vi "AutonomousGyro.vi"() -> (0 "Terminate":bool)   [LabVIEW 2015]
uses:
  <vilib>/Rock Robotics/WPI/DriverStation/WPI_DriverStationRobotMode2.ctl
  <vilib>/Rock Robotics/WPI/Solenoid/WPI_SolenoidValue.ctl
  Utilities/AutoVars.vi
  Utilities/MotorPositionGlobals.vi
  Utilities/ShiftGlobals.vi
  Utilities/VisionGlobals.vi
  Utilities/GlobalVisionVars.vi
  <vilib>/Rock Robotics/WPI/Solenoid/WPI_SolenoidSetEnum.vi
  navx-mxp/labview/navX Library v2/navX Library v2.lvlib
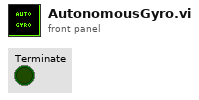
[diagram p1: front panel]
types:
  T1 = enum16{"WaitingForInput", "Driving", "TurnToTarget", "DriveMore", "Shoot", "End"}
  T2 = typedef "WPI_DriverStationRobotMode2.ctl" = enum16{"Autonomous Disabled", "Autonomous Enabled", "Teleop Disabled", "Teleop Enabled", "Disconnected", "Finish", "Test Disabled", "Test Enabled", "Emergency Stopped"}
  T3 = typedef "WPI_SolenoidValue.ctl" = enum16{"Off", "On", "Forward", "Reverse"}
  T4 = typedef "WPI_MotorControlDeviceRef.ctl" = cluster{"DeviceStatus":errorcluster, "Type":T5, "PWM":cluster{"PWM Channel":T6, "DeadBand":T7}, "CAN":cluster{"Device Number":u8, "Control Mode":T8, "Semaphore":T9, "Max Vout":dbl, "TalonSRX Control Mode":T10}, "Invert":bool}
  T5 = typedef "WPI_MotorControlType.ctl" = enum16{"PWM", "CAN", "CANTalonSRX"}
  T6 = typedef "FPGA_DIOPWMChannel.ctl" = enum8{"PWM 0", "PWM 1", "PWM 2", "PWM 3", "PWM 4", "PWM 5", "PWM 6", "PWM 7", "PWM 8", "PWM 9", "PWM MXP 0", "PWM MXP 1", "PWM MXP 2", "PWM MXP 3", "PWM MXP 4", "PWM MXP 5", "PWM MXP 6", "PWM MXP 7", "PWM MXP 8", "PWM MXP 9", "Invalid"}
  T7 = typedef "WPI_PWMDeadband.ctl" = cluster{"Name":string, "maxPositivePwm":i32, "minPositivePwm":i32, "centerPwm":i32, "maxNegativePwm":i32, "minNegativePwm":i32, "angularRange":u16}
  T8 = typedef "WPI_CANJaguar_ControlMode.ctl" = enum8{"Percent VBus", "Current", "Speed", "Position", "Voltage"}
  T9 = typedef "Semaphore RefNum" = refnum<k1>
  T10 = typedef "WPI_CANTalonSRX_APIControlMode.ctl" = enum8{"Percent VBus", "Speed", "Position", "Slave", "Unchanged / Invalid", "Voltage Compensation", "Current", "Motion Profile"}
  T11 = typedef "navX Library v2.lvlib/Z900_navX_DeviceTypeDef.ctl" = cluster{"Interface":cluster{"Protocol":T12, "Update Rate (4Hz-60Hz)":u8, "navX Open TypeDef":variant}, "Notify Packet":refnum<notifier>, "Loop VI Refnum":refnum<vi>, "Ready to Close Occurrence Refnum":refnum<k4>}
  T12 = typedef "navX Library v2.lvlib/Z900_navX_ProtocolTypeDef.ctl" = enum16{"SERIAL", "I2C", "SPI"}
  T13 = typedef "WPI_CANTalonSRX_GlobalStatus.ctl" = cluster{"Applied Throttle":dbl, "Module Enabled":bool, "CAN Error":errorcluster, "Closed Loop Error":dbl, "Forward Limit Switch Closed":bool, "Reverse Limit Switch Closed":bool, "Sensor Position":dbl, "Sensor Velocity":dbl, "Current":dbl, "Sticky Fault - Over Temp":bool, "Sticky Fault - Under Voltage":bool, "Sticky Fault - Forward Limit":bool, "Sticky Fault - Reverse Limit":bool, "Sticky Fault - Forward Soft Limit":bool, "Sticky Fault - Reverse Soft Limit":bool, "Brake is Enabled":bool, "Encoder Position":dbl, "Encoder Velocity":dbl, "Encoder Index Count":dbl, "Encoder A Pin State":bool, "Encoder B Pin State":bool, "Encoder Index Pin State":bool, "Analog In":dbl, "Analog In Velocity":dbl, "Temperature (C)":dbl, "Battery Voltage":dbl, "Control 5 Is Supported":bool, "Current Profile Slot Select":dbl, "Pos Div 8":bool, "Vel Div 4":bool, "Pulse Width Position":i32, "Pulse Width Velocity":i32, "Pulse Width Rise To Rise (us)":i32, "Pulse Width Rise To Fall (us)":i32, "Mot Prof Active Is Under Run":bool, "Mot Prof Active Has Under Run":bool, "Mot Prof Active Is Last":bool, "Mot Prof Active Velocity Only":bool, "Mot Prof Active Is Valid":bool, "Mot Prof Buffer Is Full":bool, "Mot Prof Active Profile Slot Select":i32, "Mot Prof NextID":i32, "Mot Prof Count":i32, "Mot Prof Active Velocity":dbl, "Mot Prof Active Position":dbl, "Mot Prof Output Enable":i32}
  T14 = typedef "WPI_DigitalOutputDevRef.ctl" = cluster{"DIO Channel":T15, "DevStatus":errorcluster}
  T15 = typedef "FPGA_DIOChannel.ctl" = enum8{"DIO 0", "DIO 1", "DIO 2", "DIO 3", "DIO 4", "DIO 5", "DIO 6", "DIO 7", "DIO 8", "DIO 9", "DIO MXP 0", "DIO MXP 1", "DIO MXP 2", "DIO MXP 3", "DIO MXP 4", "DIO MXP 5", "DIO MXP 6", "DIO MXP 7", "DIO MXP 8", "DIO MXP 9", "DIO MXP 10", "DIO MXP 11", "DIO MXP 12", "DIO MXP 13", "DIO MXP 14", "DIO MXP 15", "Invalid"}
  T16 = typedef "WPI_SolenoidDevRef.ctl" = cluster{"DevStatus":errorcluster, "Pneumatics Control Module":u8, "Forward Solenoid Channel":T17, "Reverse Solenoid Channel":T17}
  T17 = typedef "WPI_SolenoidChannel.ctl" = enum8{"Solenoid 0", "Solenoid 1", "Solenoid 2", "Solenoid 3", "Solenoid 4", "Solenoid 5", "Solenoid 6", "Solenoid 7", "Invalid"}
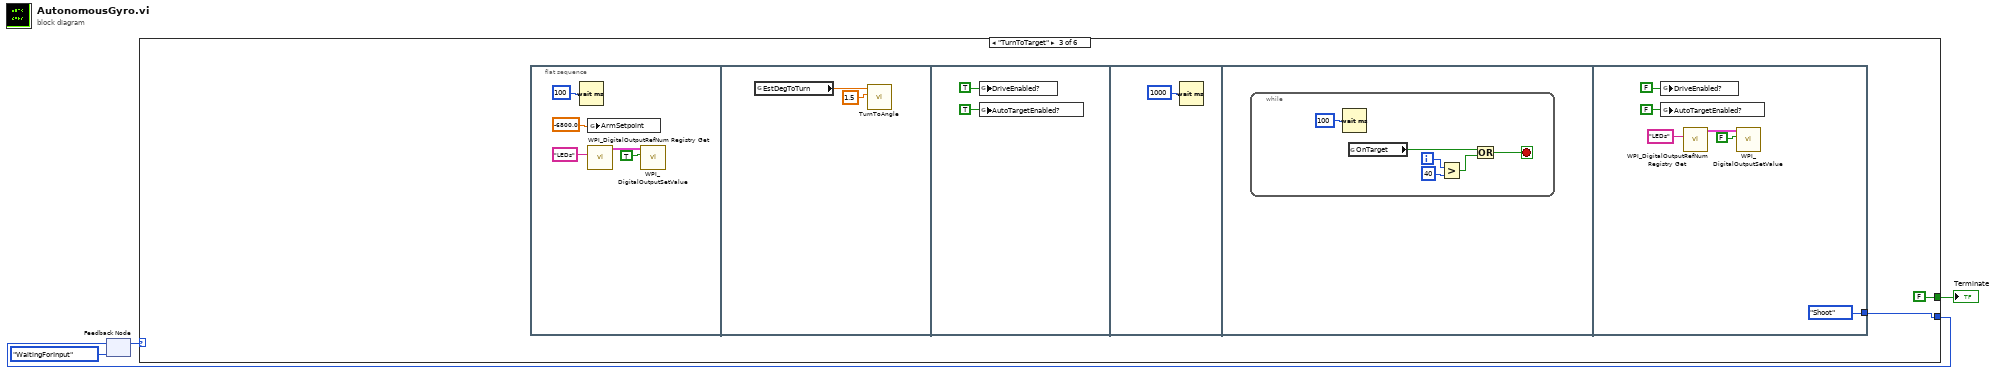
[diagram p0: block diagram]
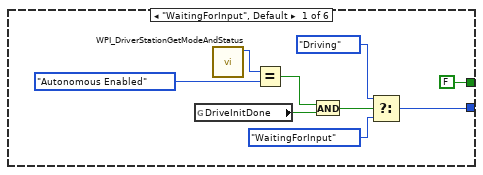
[diagram p2: hidden frame]
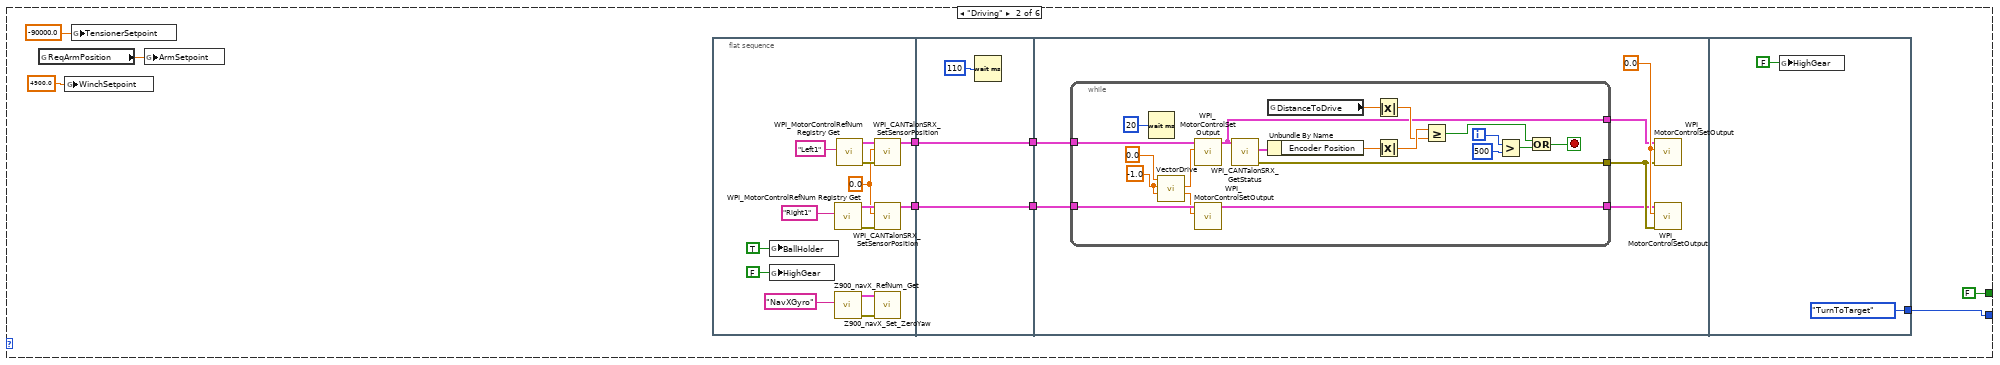
[diagram p3: hidden frame]
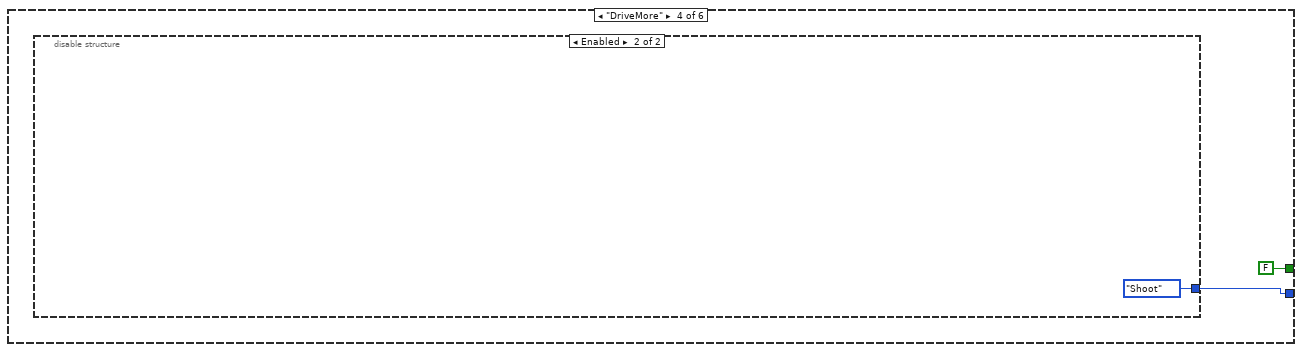
[diagram p4: hidden frame]
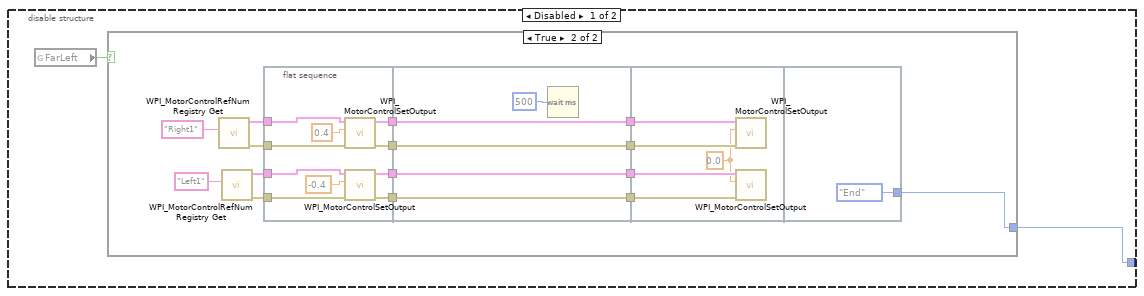
[diagram p5: hidden frame]
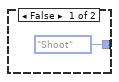
[diagram p6: hidden frame]
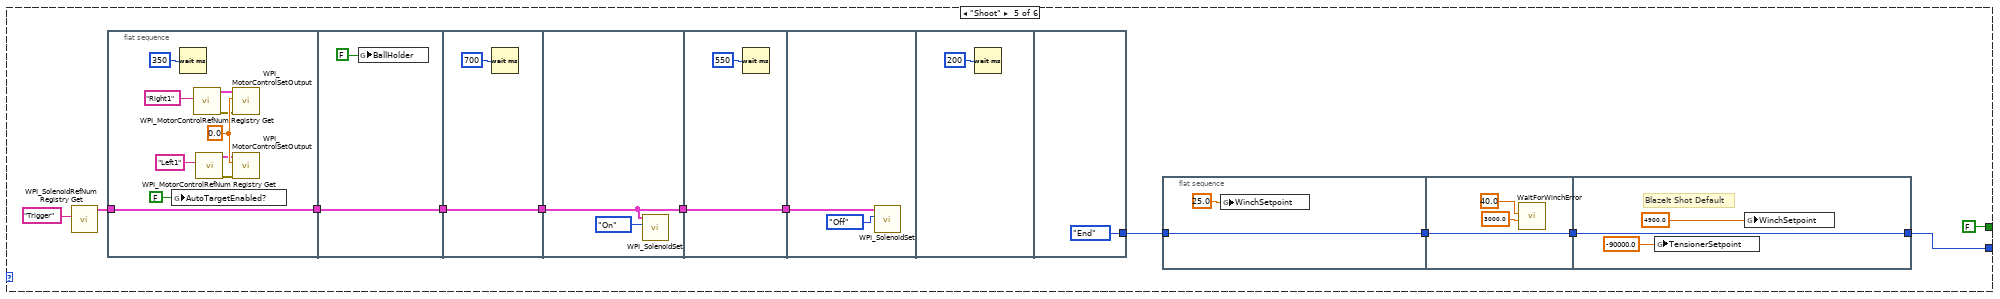
[diagram p7: hidden frame]
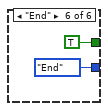
[diagram p8: hidden frame]
diagram:
  n1 = feedback #1(T1."WaitingForInput" ("AutoStateMachine")) -> (w1:T1)
  n2 = case shown="\"TurnToTarget\"" w1 {
    tunnel: [w13 w14 w69 w93 w136 T1."End" ("AutoStateMachine")] -> w4
    tunnel: [FALSE FALSE FALSE FALSE FALSE TRUE] -> w3
    frame "WaitingForInput", Default {
      n3 = global read "AutoVars.vi" "DriveInitDone"() -> (w8:bool)
      n4 = call <vilib>:"WPI_DriverStationGetModeAndStatus.vi"() -> ("Robot Mode"=w11:T2)  [unwired: 10 in, 1 out]
      n5 = Equal?(x=w11, y=WPI_DriverStationRobotMode2."Autonomous Enabled" ("Robot Mode")) -> (x = y?=w9:bool)
      n6 = And(x=w9, y=w8) -> (x .and. y?=w7:bool)
      n7 = Select(t=T1."Driving" ("AutoStateMachine"), s=w7, f=T1."WaitingForInput" ("AutoStateMachine")) -> (s? t:f=w13:T1)
    }
    frame "Driving" {
      n8 = global read "AutoVars.vi" "ReqArmPosition"() -> (w19:dbl)
      n9 = global write "MotorPositionGlobals.vi" "WinchSetpoint"(4900.0 ("WinchSetpoint")) -> ()
      n10 = global write "MotorPositionGlobals.vi" "TensionerSetpoint"(-90000.0 ("TensionerSetpoint")) -> ()
      n11 = global write "MotorPositionGlobals.vi" "ArmSetpoint"(w19) -> ()
      n12 = flat-sequence {
        tunnel: [w29] -> w18
        tunnel: [w28] -> w17
        tunnel: w18 -> [w39]
        tunnel: [w39] -> w15
        tunnel: w17 -> [w38]
        tunnel: [w38] -> w16
        tunnel: w16 -> [w43]
        tunnel: w15 -> [w42]
        tunnel: [T1."TurnToTarget" ("AutoStateMachine")] -> w14
        frame #0 {
          w30 = 0.0 ("New Sensor Position")
          n13 = global write "MotorPositionGlobals.vi" "BallHolder"(TRUE ("BallHolder")) -> ()
          n14 = global write "ShiftGlobals.vi" "HighGear"(FALSE ("HighGear")) -> ()
          n15 = call <vilib>:"WPI_MotorControlRefNum Registry Get.vi"("refnum name"="Right1") -> ("error out"=w34:errorcluster, "MotorControlDevRef"=w33:T4)  [unwired: 9 in]
          n16 = call "Z900_navX_RefNum_Get.vi"("refnum name"="NavXGyro") -> ("error out"=w25:errorcluster, "navX Device"=w26:T11)  [unwired: 9 in]
          n17 = call <vilib>:"WPI_MotorControlRefNum Registry Get.vi"("refnum name"="Left1") -> ("error out"=w32:errorcluster, "MotorControlDevRef"=w31:T4)  [unwired: 9 in]
          n18 = call <vilib>:"WPI_CANTalonSRX_SetSensorPosition.vi"("error in (no error)"=w32, "New Sensor Position"=w30, "CAN Talon SRX Ref"=w31) -> ("CAN Talon SRX Ref"=w28:T4)  [unwired: 7 in, 1 out]
          n19 = call <vilib>:"WPI_CANTalonSRX_SetSensorPosition.vi"("error in (no error)"=w34, "New Sensor Position"=w30, "CAN Talon SRX Ref"=w33) -> ("CAN Talon SRX Ref"=w29:T4)  [unwired: 7 in, 1 out]
          n20 = call "Z900_navX_Set_ZeroYaw.vi"("error in (no error)"=w25, "navX Device"=w26) -> ()  [unwired: 8 in, 2 out]
        }
        frame #1 {
          n21 = Wait (ms)(milliseconds to wait=u32 110) -> ()  [unwired: 1 out]
        }
        frame #2 {
          w45 = 0.0 ("Output")
          n22 = while {
            tunnel: [w55] -> w44
            tunnel: w43 -> [w54]
            tunnel: w42 -> [w53]
            tunnel: [w52] -> w41
            tunnel: [w51] -> w40
            i -> [w60]
            stop <- w62 stop-if-true
            w48 = -1.0 ("Output")
            n23 = Wait (ms)(milliseconds to wait=u32 20) -> ()  [unwired: 1 out]
            n24 = call "VectorDrive.vi"("RightMotorInput"=w48, "LeftMotorInput"=w48, "setpoint"=0.0) -> ("RightMotorOutput"=w49:dbl, "LeftMotorOutput"=w50:dbl)  [unwired: 7 in]
            n25 = call <vilib>:"WPI_MotorControlSetOutput.vi"("Output"=w50, "MotorControlDevRef"=w54) -> ("MotorControlDevRef"=w52:T4)  [unwired: 7 in, 2 out]
            n26 = call <vilib>:"WPI_MotorControlSetOutput.vi"("Output"=w49, "MotorControlDevRef"=w53) -> ("MotorControlDevRef"=w51:T4)  [unwired: 7 in, 2 out]
            n27 = call <vilib>:"WPI_CANTalonSRX_GetStatus.vi"("CAN Talon SRX Ref"=w52) -> ("error out"=w55:errorcluster, "Talon SRX Status"=w64:T13)  [unwired: 8 in, 1 out]
            n28 = global read "AutoVars.vi" "DistanceToDrive"() -> (w46:dbl)
            n29 = Unbundle By Name(w64) -> ("Encoder Position"=w58:dbl)
            n30 = Absolute Value(x=w46) -> (abs(x)=w56:dbl)
            n31 = Absolute Value(x=w58) -> (abs(x)=w57:dbl)
            n32 = Greater Or Equal?(x=w57, y=w56) -> (x >= y?=w63:bool)
            n33 = Greater?(x=w60, y=500) -> (0:w61:bool)
            n34 = Or(x=w63, y=w61) -> (x .or. y?=w62:bool)
          }
          n35 = call <vilib>:"WPI_MotorControlSetOutput.vi"("error in (no error)"=w44, "Output"=w45, "MotorControlDevRef"=w41) -> ()  [unwired: 6 in, 3 out]
          n36 = call <vilib>:"WPI_MotorControlSetOutput.vi"("error in (no error)"=w44, "Output"=w45, "MotorControlDevRef"=w40) -> ()  [unwired: 6 in, 3 out]
        }
        frame #3 {
          n37 = global write "ShiftGlobals.vi" "HighGear"(FALSE ("HighGear")) -> ()
        }
      }
    }
    frame "TurnToTarget" {
      n38 = flat-sequence {
        tunnel: [T1."Shoot" ("AutoStateMachine")] -> w69
        frame #0 {
          n39 = Wait (ms)(milliseconds to wait=u32 100) -> ()  [unwired: 1 out]
          n40 = global write "MotorPositionGlobals.vi" "ArmSetpoint"(-6800.0 ("ArmSetpoint")) -> ()
          n41 = call <vilib>:"WPI_DigitalOutputRefNum Registry Get.vi"("refnum name"="LEDs") -> ("DigitalOutputDevRef"=w72:T14)  [unwired: 9 in, 1 out]
          n42 = call <vilib>:"WPI_DigitalOutputSetValue.vi"("Value"=TRUE, "DigitalOutputDevRef"=w72) -> ()  [unwired: 8 in, 2 out]
        }
        frame #1 {
          n43 = global read "AutoVars.vi" "EstDegToTurn"() -> (w76:dbl)
          n44 = call "TurnToAngle.vi"("AllowedDeviation"=1.5, "GyroValue"=w76) -> ()  [unwired: 10 in]
        }
        frame #2 {
          n45 = global write "VisionGlobals.vi" "DriveEnabled?"(TRUE ("DriveEnabled?")) -> ()
          n46 = global write "VisionGlobals.vi" "AutoTargetEnabled?"(TRUE ("AutoTargetEnabled?")) -> ()
        }
        frame #3 {
          n47 = Wait (ms)(milliseconds to wait=u32 1000) -> ()  [unwired: 1 out]
        }
        frame #4 {
          n48 = while {
            i -> [w82]
            stop <- w83 stop-if-true
            n49 = Wait (ms)(milliseconds to wait=u32 100) -> ()  [unwired: 1 out]
            n50 = global read "GlobalVisionVars.vi" "OnTarget"() -> (w84:bool)
            n51 = Greater?(x=w82, y=40) -> (0:w80:bool)
            n52 = Or(x=w84, y=w80) -> (x .or. y?=w83:bool)
          }
        }
        frame #5 {
          n53 = global write "VisionGlobals.vi" "DriveEnabled?"(FALSE ("DriveEnabled?")) -> ()
          n54 = global write "VisionGlobals.vi" "AutoTargetEnabled?"(FALSE ("AutoTargetEnabled?")) -> ()
          n55 = call <vilib>:"WPI_DigitalOutputRefNum Registry Get.vi"("refnum name"="LEDs") -> ("DigitalOutputDevRef"=w89:T14)  [unwired: 9 in, 1 out]
          n56 = call <vilib>:"WPI_DigitalOutputSetValue.vi"("Value"=FALSE, "DigitalOutputDevRef"=w89) -> ()  [unwired: 8 in, 2 out]
        }
      }
    }
    frame "DriveMore" {
      n57 = disable-structure shown="Enabled" {
        disable-tunnel: [w95 T1."Shoot" ("AutoStateMachine")] -> w93
        frame Disabled {
          n58 = global read "AutoVars.vi" "FarLeft"() -> (w94:bool)
          n59 = case shown="True" w94 {
            tunnel: [T1."Shoot" ("AutoStateMachine") w109] -> w95
            frame False {
            }
            frame True {
              n60 = call <vilib>:"WPI_MotorControlRefNum Registry Get.vi"("refnum name"="Right1") -> ("error out"=w105:errorcluster, "MotorControlDevRef"=w106:T4)  [unwired: 9 in]
              n61 = call <vilib>:"WPI_MotorControlRefNum Registry Get.vi"("refnum name"="Left1") -> ("error out"=w107:errorcluster, "MotorControlDevRef"=w108:T4)  [unwired: 9 in]
              n62 = flat-sequence {
                tunnel: w108 -> [w121]
                tunnel: w107 -> [w120]
                tunnel: w106 -> [w119]
                tunnel: w105 -> [w118]
                tunnel: [w117] -> w104
                tunnel: [w116] -> w103
                tunnel: [w115] -> w102
                tunnel: [w114] -> w98
                tunnel: w104 -> [w124]
                tunnel: w103 -> [w122]
                tunnel: w102 -> [w125]
                tunnel: [w125] -> w101
                tunnel: [w124] -> w100
                tunnel: [w123] -> w99
                tunnel: w98 -> [w123]
                tunnel: [w122] -> w97
                tunnel: w101 -> [w131]
                tunnel: w100 -> [w130]
                tunnel: w99 -> [w129]
                tunnel: w97 -> [w128]
                tunnel: [T1."End" ("AutoStateMachine")] -> w109
                frame #0 {
                  n63 = call <vilib>:"WPI_MotorControlSetOutput.vi"("error in (no error)"=w118, "Output"=0.4, "MotorControlDevRef"=w119) -> ("error out"=w117:errorcluster, "MotorControlDevRef"=w115:T4)  [unwired: 6 in, 1 out]
                  n64 = call <vilib>:"WPI_MotorControlSetOutput.vi"("error in (no error)"=w120, "Output"=-0.4, "MotorControlDevRef"=w121) -> ("error out"=w116:errorcluster, "MotorControlDevRef"=w114:T4)  [unwired: 6 in, 1 out]
                }
                frame #1 {
                  n65 = Wait (ms)(milliseconds to wait=u32 500) -> ()  [unwired: 1 out]
                }
                frame #2 {
                  w127 = 0.0 ("Output")
                  n66 = call <vilib>:"WPI_MotorControlSetOutput.vi"("error in (no error)"=w130, "Output"=w127, "MotorControlDevRef"=w131) -> ()  [unwired: 6 in, 3 out]
                  n67 = call <vilib>:"WPI_MotorControlSetOutput.vi"("error in (no error)"=w128, "Output"=w127, "MotorControlDevRef"=w129) -> ()  [unwired: 6 in, 3 out]
                }
                frame #3 {
                }
              }
            }
          }
        }
        frame Enabled {
        }
      }
    }
    frame "Shoot" {
      n68 = call <vilib>:"WPI_SolenoidRefNum Registry Get.vi"("refnum name"="Trigger") -> ("SolenoidDevRef"=w141:T16)  [unwired: 9 in, 1 out]
      n69 = flat-sequence {
        tunnel: [w163] -> w135
        tunnel: w141 -> [w163]
        tunnel: w135 -> [w165]
        tunnel: [w165] -> w134
        tunnel: w134 -> [w167]
        tunnel: [w167] -> w145
        tunnel: [w168] -> w144
        tunnel: w145 -> [w168]
        tunnel: w144 -> [w170]
        tunnel: [w170] -> w143
        tunnel: w143 -> [w172]
        tunnel: [T1."End" ("AutoStateMachine")] -> w139
        frame #0 {
          w158 = 0.0
          n70 = global write "VisionGlobals.vi" "AutoTargetEnabled?"(FALSE ("AutoTargetEnabled?")) -> ()
          n71 = Wait (ms)(milliseconds to wait=u32 350) -> ()  [unwired: 1 out]
          n72 = call <vilib>:"WPI_MotorControlRefNum Registry Get.vi"("refnum name"="Right1") -> ("error out"=w156:errorcluster, "MotorControlDevRef"=w157:T4)  [unwired: 9 in]
          n73 = call <vilib>:"WPI_MotorControlRefNum Registry Get.vi"("refnum name"="Left1") -> ("error out"=w154:errorcluster, "MotorControlDevRef"=w155:T4)  [unwired: 9 in]
          n74 = call <vilib>:"WPI_MotorControlSetOutput.vi"("error in (no error)"=w156, "Output"=w158, "MotorControlDevRef"=w157) -> ()  [unwired: 6 in, 3 out]
          n75 = call <vilib>:"WPI_MotorControlSetOutput.vi"("error in (no error)"=w154, "Output"=w158, "MotorControlDevRef"=w155) -> ()  [unwired: 6 in, 3 out]
        }
        frame #1 {
          n76 = global write "MotorPositionGlobals.vi" "BallHolder"(FALSE ("BallHolder")) -> ()
        }
        frame #2 {
          n77 = Wait (ms)(milliseconds to wait=u32 700) -> ()  [unwired: 1 out]
        }
        frame #3 {
          n78 = call-poly <vilib>:"WPI_SolenoidSet.vi"("Value"=WPI_SolenoidValue."On", "SolenoidDevRef"=w168) -> ()  [unwired: 8 in, 2 out]
        }
        frame #4 {
          n79 = Wait (ms)(milliseconds to wait=u32 550) -> ()  [unwired: 1 out]
        }
        frame #5 {
          n80 = call-poly <vilib>:"WPI_SolenoidSet.vi"("Value"=WPI_SolenoidValue."Off", "SolenoidDevRef"=w172) -> ()  [unwired: 8 in, 2 out]
        }
        frame #6 {
          n81 = Wait (ms)(milliseconds to wait=u32 200) -> ()  [unwired: 1 out]
        }
        frame #7 {
        }
      }
      n82 = flat-sequence {
        tunnel: w139 -> [w146]
        tunnel: [w146] -> w137
        tunnel: [w148] -> w138
        tunnel: w137 -> [w148]
        tunnel: [w151] -> w136
        tunnel: w138 -> [w151]
        frame #0 {
          n83 = global write "MotorPositionGlobals.vi" "WinchSetpoint"(25.0 ("WinchPosition")) -> ()
        }
        frame #1 {
          n84 = call "WaitForWinchError.vi"("Timeout (ms)"=3000.0, "AllowedError"=40.0) -> ()  [unwired: 9 in, 1 out]
        }
        frame #2 {
          # "BlazeIt Shot Default"
          n85 = global write "MotorPositionGlobals.vi" "TensionerSetpoint"(-90000.0 ("TensionerSetpoint")) -> ()
          n86 = global write "MotorPositionGlobals.vi" "WinchSetpoint"(4900.0 ("WinchPosition")) -> ()
        }
      }
    }
    frame "End" {
    }
  }
  "Terminate" <- w3
  n87 = feedback-in #1(w4) -> ()
